vi "JoyMath.vi"(11 "input cluster":T1) -> (0 "Y axis 2":fxp<+/-,9,2> format="%#.2g", 1 "X axis 2":fxp<+/-,9,2> format="%#.2g", 2 "Y axis 1":fxp<+/-,9,2> format="%#.2g", 3 "X axis 1":fxp<+/-,9,2>, 5 "Triggers":fxp<+/-,9,2> format="%#.2g")   [LabVIEW 2012]
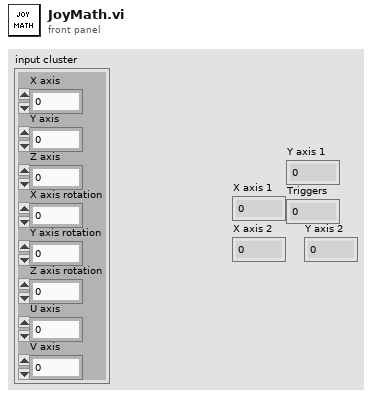
[diagram p1: front panel]
types:
  T1 = cluster{"X axis":i32, "Y axis":i32, "Z axis":i32, "X axis rotation":i32, "Y axis rotation":i32, "Z axis rotation":i32, "U axis":i32, "V axis":i32}
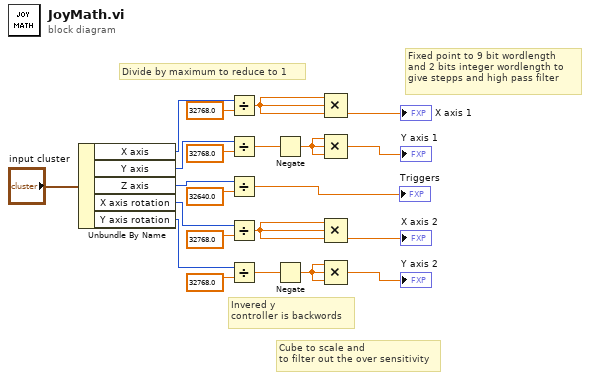
[diagram p0: block diagram]
diagram:
  # "Fixed point to 9 bit wordlength\nand 2 bits integer wordlength to \ngive stepps and high pass filter"
  # "Invered y\ncontroller is backwords"
  # "Divide by maximum to reduce to 1"
  # "Cube to scale and\nto filter out the over sensitivity"
  n1 = Unbundle By Name("input cluster") -> ("X axis"=w5:i32, "Y axis"=w6:i32, "Z axis"=w15:i32, "X axis rotation"=w9:i32, "Y axis rotation"=w12:i32)
  n2 = Divide(x=w5, y=sgl 32768.0) -> (x/y=w3:sgl)
  n3 = Divide(x=w6, y=sgl 32768.0) -> (x/y=w4:sgl)
  n4 = Divide(x=w15, y=sgl 32640.0) -> (x/y=→"Triggers":sgl)
  n5 = Divide(x=w9, y=sgl 32768.0) -> (x/y=w10:sgl)
  n6 = Divide(x=w12, y=sgl 32768.0) -> (x/y=w14:sgl)
  n7 = Negate(x=w4) -> (-x=w21:sgl)
  n8 = Negate(x=w14) -> (-x=w18:sgl)
  n9 = Compound Arithmetic op=MULTIPLY(w3, w3, w3) -> (→"X axis 1":sgl)
  n10 = Compound Arithmetic op=MULTIPLY(w21, w21, w21) -> (→"Y axis 1":sgl)
  n11 = Compound Arithmetic op=MULTIPLY(w10, w10, w10) -> (→"X axis 2":sgl)
  n12 = Compound Arithmetic op=MULTIPLY(w18, w18, w18) -> (→"Y axis 2":sgl)
